vi "Tx Packet Page.vi"(8 "error in (no error)":errorcluster, 11 "Node Ptr":T3 format="%.0x") -> (0 "error out":errorcluster)   [LabVIEW 2019, in "UDP-Custom-Device System Explorer.lvlib"]
uses:
  UDP-Custom-Device System Explorer.lvlib
  Shared/Types/Shared - Transmit Flag Options.ctl
  Shared/Types/Shared - Transmit Echo Options.ctl
  <vilib>/NI VeriStand/Custom Device API/Custom Device Item Ref.ctl
  Types/Page References/Refs - Tx Packets Page.ctl
  Shared/Types/Shared - Channel Data Type.ctl
  <vilib>/NI VeriStand/Custom Device API/Custom Device API.lvlib
  Property Accessors/Tx Packet Accessors.lvlib
  Shared/UDP-Custom-Device Shared.lvlib
  <vilib>/NI VeriStand/Custom Device Tools/Custom Device Utility Library/Custom Device Utility Library.lvlib
  Property Accessors/Shared Packet Accessors.lvlib
  Property Accessors/Tx Channel Accessors.lvlib
  Property Accessors/Tx Channel Section Accessors.lvlib
panel:
  in  "Config Threading":bool
  in  "Debug Mode":bool caption="Auto-Assign Local NIC"
  in  "Transmit Echo Options":T1
  in  "Transmit Options":T2=enum."One-Shot"
  in  "Port as Channel?":bool caption="Auto-Assign Local NIC"
  in  "TTL":u16=1
  in  "Multicast?":bool caption="Auto-Assign Local NIC"
  in  "Channel Config Export":bool
  in  "Configure Header":bool
  in  "Endianness":u16(ring) items=["big-endian"=0, "little-endian"=2]
  in  "Auto-Assign Local NIC":bool
  in  "Port":u16
  in  "IP Address of Local NIC":string
  in  "General Header 3":cluster{"Section Name":string}={"Section Name"="Network Settings"}
  out "Packet ID":i32
  in  "Destination Port":u16
  in  "IP Address of Destination":string
  in  "Description":string
  in  "Name":string
  in  "General Header 2":cluster{"Section Name":string}={"Section Name"="Configured Channels"}
  in  "Tx Channels":i32[](listbox)
  in  "SHDocVw.IWebBrowser":refnum<k7>(container)
  in  "General Header":cluster{"Section Name":string}={"Section Name"="Packet Configuration"}
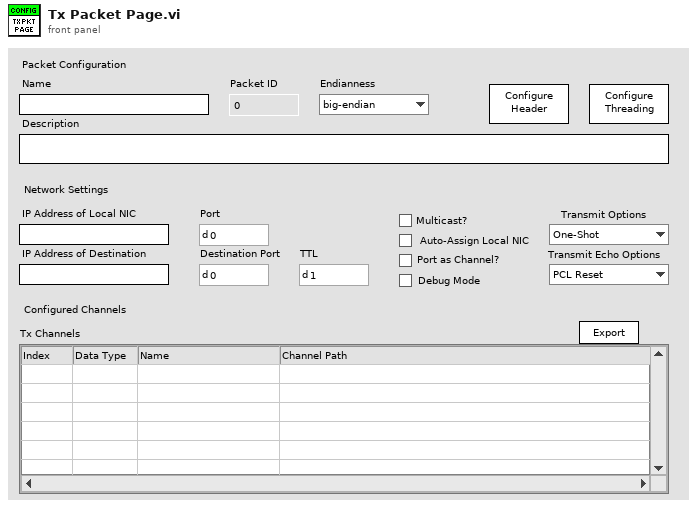
[diagram p1: front panel]
types:
  T1 = typedef "UDP-Custom-Device Shared.lvlib/Shared - Transmit Echo Options.ctl" = enum16{"PCL Reset", "Counter", "Mirror"}
  T2 = typedef "UDP-Custom-Device Shared.lvlib/Shared - Transmit Flag Options.ctl" = enum16{"Always", "One-Shot", "Toggle"}
  T3 = typedef "Custom Device API.lvlib/Custom Device Item Ref.ctl" = u64
  T4 = typedef "UDP-Custom-Device System Explorer.lvlib/Refs - Tx Packets Page.ctl" = cluster{"Tx Channels":refnum<vi>, "Name":refnum<vi>, "Description":refnum<vi>, "Packet ID":refnum<vi>, "Dest IP Address":refnum<vi>, "Dest Port":refnum<vi>, "Source IP Address":refnum<vi>, "Source Port":refnum<vi>, "Auto Assign Local NIC":refnum<vi>, "Endianness":refnum<vi>, "Channel Config Export":refnum<vi>, "TTL":refnum<vi>, "Multicast?":refnum<vi>, "Port as Channel?":refnum<vi>, "Transmit Options":refnum<vi>, "Transmit Echo Options":refnum<vi>, "Debug Mode":refnum<vi>}
  T5 = enum8{"Enabled", "Disabled", "Disabled and Grayed Out"}
  T6 = typedef "UDP-Custom-Device Shared.lvlib/Shared - Channel Data Type.ctl" = enum16{"Boolean", "Single", "Double", "I8", "I16", "I32", "I64", "U8", "U16", "U32", "U64"}
  T7 = typedef "Custom Device API.lvlib/Custom Device Commands.ctl" = enum16{"Default", "Item renamed", "Shutdown", "Dynamic button pressed"}
  T8 = typedef "UDP-Custom-Device System Explorer.lvlib/Thread Configuration.ctl" = cluster{"targetProcessor":i8, "targetPriority":i16, "Synchronization":T9, "loopPeriod":u32, "pclDecimation":u16, "threadManagement":T10}
  T9 = typedef "UDP-Custom-Device System Explorer.lvlib/Thread Sync Reference.ctl" = enum16{"PCL", "Async"}
  T10 = typedef "UDP-Custom-Device Shared.lvlib/Shared - Thread Management.ctl" = enum16{"Untimed (Default)", "Timed (High Priority)"}
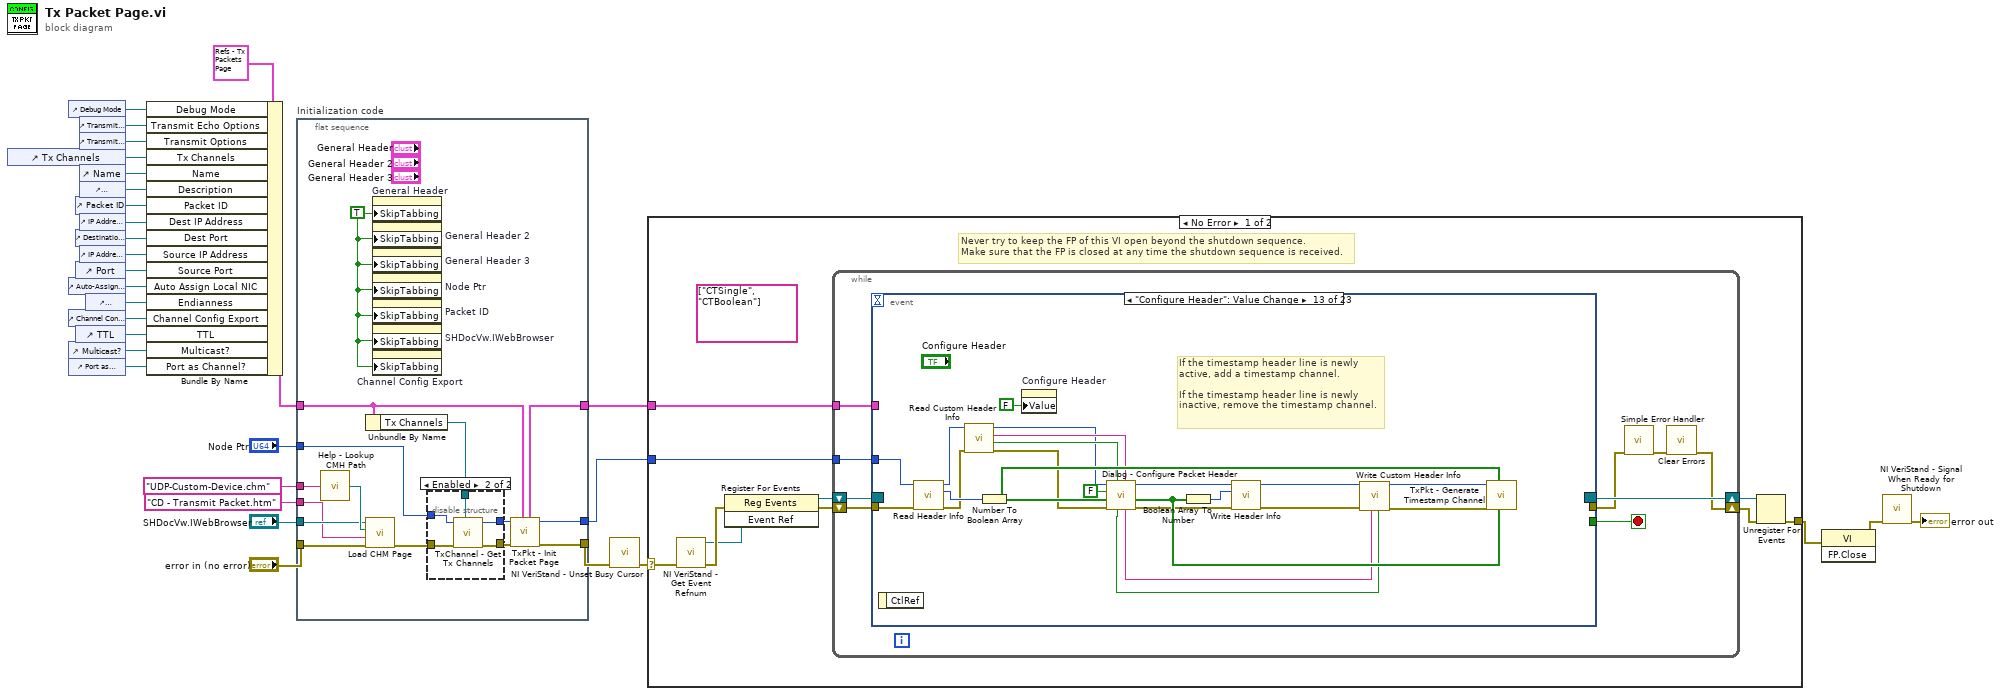
[diagram p0: block diagram]
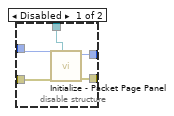
[diagram p2: hidden frame]
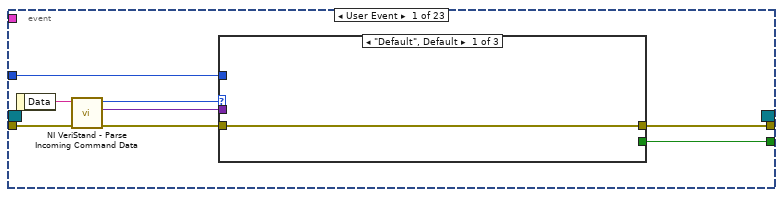
[diagram p3: hidden frame]
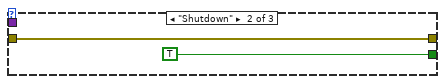
[diagram p4: hidden frame]
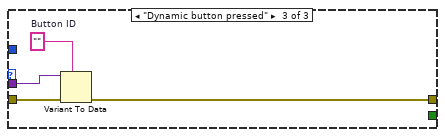
[diagram p5: hidden frame]
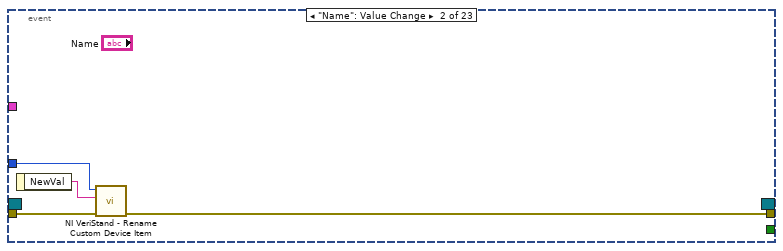
[diagram p6: hidden frame]
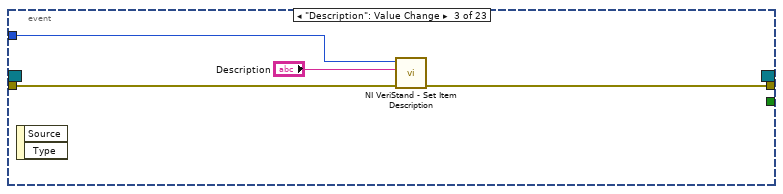
[diagram p7: hidden frame]
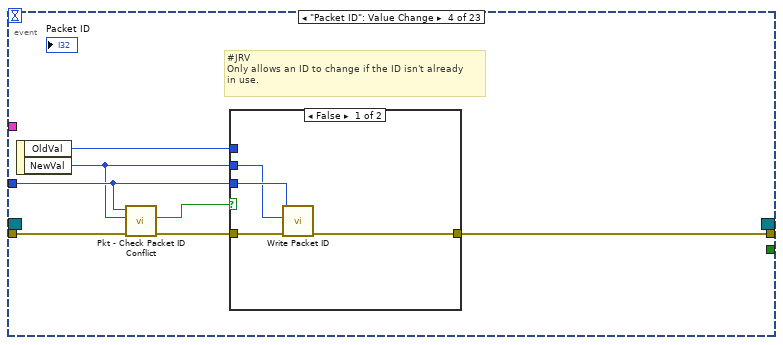
[diagram p8: hidden frame]
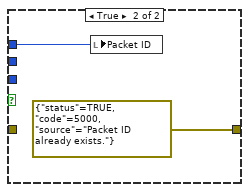
[diagram p9: hidden frame]
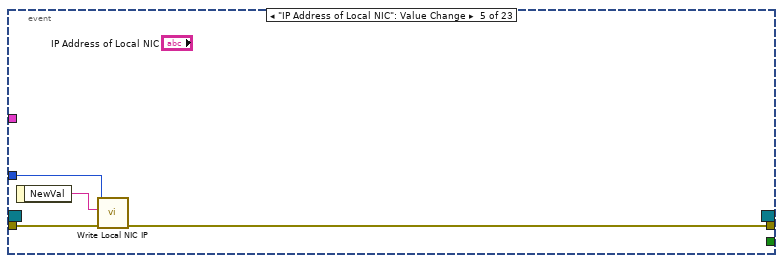
[diagram p10: hidden frame]
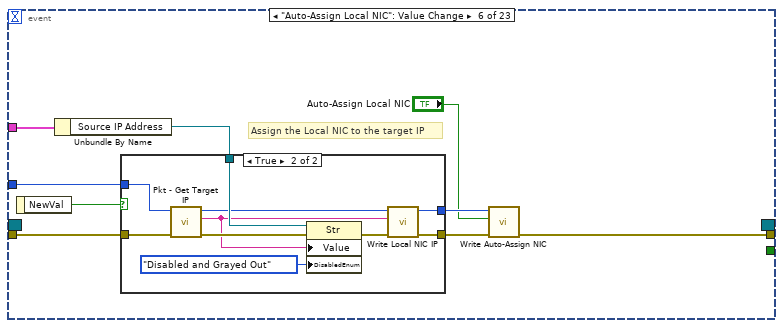
[diagram p11: hidden frame]
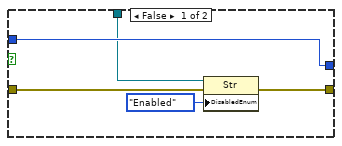
[diagram p12: hidden frame]
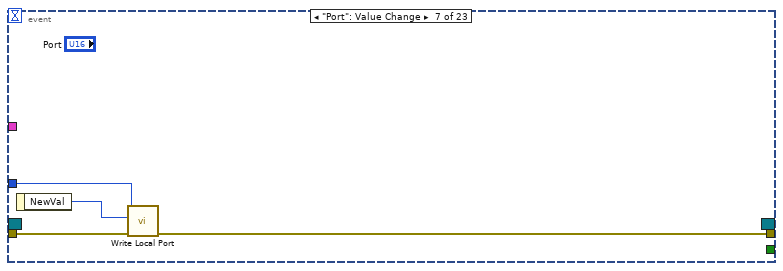
[diagram p13: hidden frame]
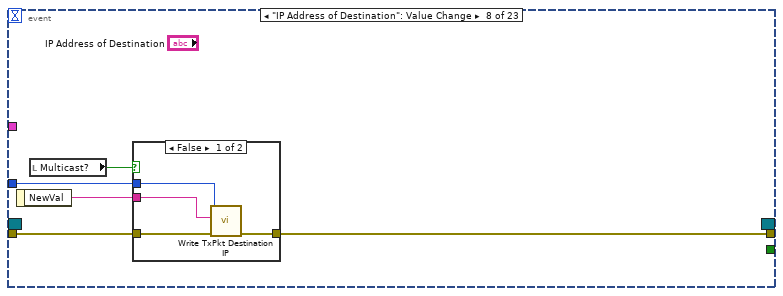
[diagram p14: hidden frame]
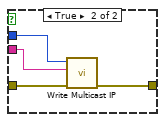
[diagram p15: hidden frame]
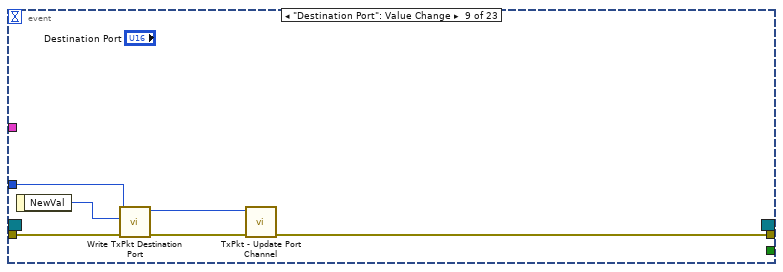
[diagram p16: hidden frame]
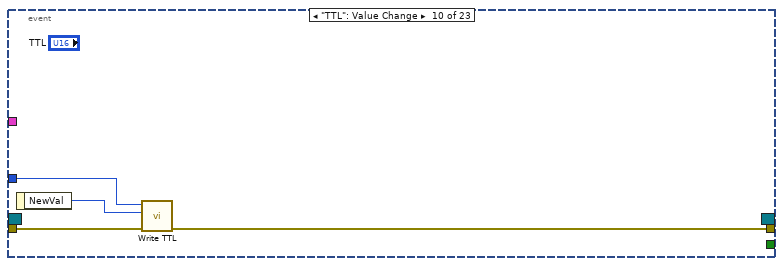
[diagram p17: hidden frame]
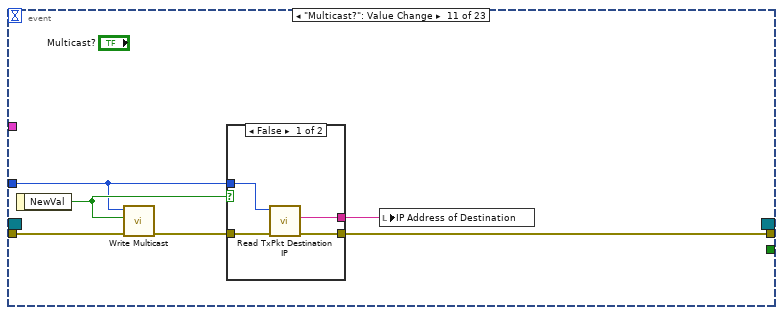
[diagram p18: hidden frame]
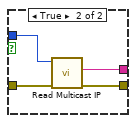
[diagram p19: hidden frame]
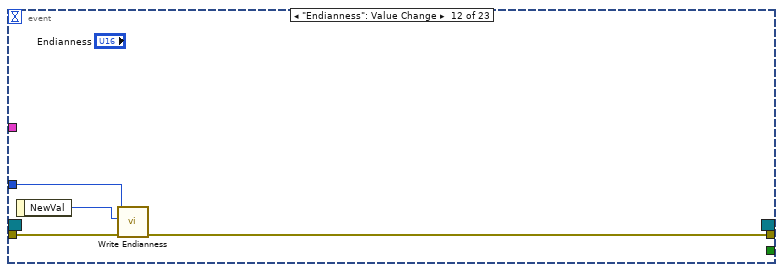
[diagram p20: hidden frame]
diagram:
  n1 = control-ref of="Tx Channels"() -> (w17:refnum<vi>)
  n2 = control-ref of="Debug Mode"() -> (w1:refnum<vi>)
  n3 = control-ref of="Auto-Assign Local NIC"() -> (w10:refnum<vi>)
  n4 = control-ref of="Channel Config Export"() -> (w7:refnum<vi>)
  n5 = control-ref of="Multicast?"() -> (w5:refnum<vi>)
  n6 = control-ref of="Port as Channel?"() -> (w4:refnum<vi>)
  n7 = control-ref of="Packet ID"() -> (w13:refnum<vi>)
  n8 = control-ref of="Destination Port"() -> (w14:refnum<vi>)
  n9 = control-ref of="Port"() -> (w11:refnum<vi>)
  n10 = control-ref of="TTL"() -> (w6:refnum<vi>)
  n11 = control-ref of="Transmit Echo Options"() -> (w2:refnum<vi>)
  n12 = control-ref of="Transmit Options"() -> (w3:refnum<vi>)
  n13 = control-ref of="Name"() -> (w9:refnum<vi>)
  n14 = control-ref of="Description"() -> (w16:refnum<vi>)
  n15 = control-ref of="IP Address of Destination"() -> (w15:refnum<vi>)
  n16 = control-ref of="IP Address of Local NIC"() -> (w12:refnum<vi>)
  n17 = control-ref of="Endianness"() -> (w8:refnum<vi>)
  n18 = Bundle By Name(cluster=T4 {"Tx Channels"=refnum, "Name"=refnum, "Description"=refnum, "Packet ID"=refnum, "Dest IP Address"=refnum, "Dest Port"=refnum, "Source IP Address"=refnum, "Source Port"=refnum, "Auto Assign Local NIC"=refnum, "Endianness"=refnum, "Channel Config Export"=refnum, "TTL"=refnum, "Multicast?"=refnum, "Port as Channel?"=refnum, "Transmit Options"=refnum, "Transmit Echo Options"=refnum, "Debug Mode"=refnum} ("Tx Channels Section Cluster"), "Debug Mode"=w1, "Transmit Echo Options"=w2, "Transmit Options"=w3, "Tx Channels"=w17, "Name"=w9, "Description"=w16, "Packet ID"=w13, "Dest IP Address"=w15, "Dest Port"=w14, "Source IP Address"=w12, "Source Port"=w11, "Auto Assign Local NIC"=w10, "Endianness"=w8, "Channel Config Export"=w7, "TTL"=w6, "Multicast?"=w5, "Port as Channel?"=w4) -> (w20:T4)
  n19 = flat-sequence "Initialization code" {
    tunnel: "error in (no error)" -> [w37]
    tunnel: "Node Ptr" -> [w46]
    tunnel: [w41] -> w27
    tunnel: [w42] -> w24
    tunnel: "SHDocVw.IWebBrowser" -> [w36]
    tunnel: "CD - Transmit Packet.htm" ("CD_CHM_Section") -> [w34]
    tunnel: "UDP-Custom-Device.chm" ("CD_CHM_FileName") -> [w35]
    tunnel: w20 -> [w40]
    tunnel: [w39] -> w19
    frame #0 {
      w32 = TRUE ("Skip When Tabbing")
      n20 = call "Help - Lookup CMH Path.vi"("Main CMH File"=w35) -> ("Compiled CMH Path"=w38:path)
      n21 = Unbundle By Name(w40) -> ("Tx Channels"=w45:refnum<vi>)
      n22 = call <vilib>:"Load CHM Page.vi"("error in (no error)"=w37, "HTML File"=w34, "Compiled CHM Path"=w38, "Web Browser Reference"=w36) -> ("error out"=w33:errorcluster)  [unwired: 7 in]
      n23 = property on="General Header" class="Clust (strict)"("SkipTabbing"=w32) -> ()  [unwired: 2 in, 2 out]
      n24 = property on="General Header 2" class="Clust (strict)"("SkipTabbing"=w32) -> ()  [unwired: 2 in, 2 out]
      n25 = property on="General Header 3" class="Clust (strict)"("SkipTabbing"=w32) -> ()  [unwired: 2 in, 2 out]
      n26 = property on="Node Ptr" class="DigNum (strict)"("SkipTabbing"=w32) -> ()  [unwired: 2 in, 2 out]
      n27 = property on="Packet ID" class="DigNum (strict)"("SkipTabbing"=w32) -> ()  [unwired: 2 in, 2 out]
      n28 = property on="SHDocVw.IWebBrowser" class="AXCont"("SkipTabbing"=w32) -> ()  [unwired: 2 in, 2 out]
      n29 = property on="Channel Config Export" class="Bool"("SkipTabbing"=w32) -> ()  [unwired: 2 in, 2 out]
      n30 = disable-structure shown="Enabled" {
        disable-tunnel: w46 -> [w51 w55]
        disable-tunnel: w45 -> [w50 w54]
        disable-tunnel: [w49 w52] -> w44
        disable-tunnel: [w48 w53] -> w43
        disable-tunnel: w33 -> [w47 w56]
        frame Disabled {
          n31 = call "Initialize - Packet Page Panel.vi"("Channels Listbox"=w50, "error in (no error)"=w47, "Item Ref in"=w51) -> ("error out"=w49:errorcluster, "Item Ref out"=w48:T3)  [unwired: 7 in]
        }
        frame Enabled {
          n32 = call "TxChannel - Get Tx Channels.vi"("MCLB"=w54, "error in (no error)"=w56, "Node Ptr"=w55) -> ("error out"=w52:errorcluster, "Node Ptr out"=w53:T3)  [unwired: 6 in, 1 out]
        }
      }
      n33 = call "TxPkt - Init Packet Page.vi"("Tx Packets Cluster In"=w40, "error in (no error)"=w44, "Node Ptr In"=w43) -> ("error out"=w41:errorcluster, "Node Ptr Out"=w42:T3, "Tx Packets Cluster Out"=w39:T4)  [unwired: 6 in]
    }
  }
  n34 = call <vilib>:"NI VeriStand - Unset Busy Cursor.vi"("error in (no error)"=w27) -> ("error out"=w26:errorcluster)  [unwired: 10 out]
  n35 = case shown="No Error" w26 {
    selector: w26 -> [w58 w343]
    tunnel: [w63 w341] -> w31
    tunnel: w24 -> [w59 _]
    tunnel: w19 -> [w57 _]
    frame No Error {
      (unwired) string[] ["CTSingle", "CTBoolean"] ("item names")
      # "Never try to keep the FP of this VI open beyond the shutdown sequence.\nMake sure that the FP is closed at any time the shutdown sequence is received."
      n36 = call <vilib>:"NI VeriStand - Get Event Refnum.vi"("error in (no error)"=w58) -> ("error out"=w66:errorcluster, "Event Ref"=w62:refnum<user-event>)  [unwired: 9 out]
      n37 = register-events(error in=w66, w62) -> (reference out=w60:refnum<event-registration>, error out=w61:errorcluster)  [unwired: 1 in]
      n38 = while {
        tunnel: w59 -> [w71]
        shift-right: [w68] -> w64
        shift-left: w61 -> [w74]
        shift-right: [w75] -> w65
        shift-left: w60 -> [w73]
        tunnel: w57 -> [w67]
        stop <- w72 stop-if-true
        n39 = event shown="[12] \"Configure Header\": Value Change" {
          selector: w73 -> [_ _ _ _ _ _ _ _ _ _ _ _ _ _ _ _ _ _ _ _ _ _ _]
          dyn-events: [_ _ _ _ _ _ _ _ _ _ _ _ _ _ _ _ _ _ _ _ _ _ _] -> w75
          timeout: _ -> [_ _ _ _ _ _ _ _ _ _ _ _ _ _ _ _ _ _ _ _ _ _ _]
          tunnel: w74 -> [w83 w94 w98 w100 w114 w124 w142 w148 w160 w164 w172 w184 w200 w213 w223 w226 w230 w233 w241 w245 w275 _ w287]
          tunnel: [w79 _ _ _ _ _ _ _ _ _ _ _ _ _ _ _ _ _ _ _ _ _ _] -> w72
          tunnel: [w78 w91 w95 w105 w113 w117 w141 w145 w157 w163 w170 w183 _ w209 w219 w224 w229 w232 w236 w244 w253 _ w286] -> w70
          tunnel: w71 -> [w77 w92 w97 w103 w115 w123 w143 w147 w162 w166 w167 w182 w201 w217 w222 w227 w231 w235 w242 w246 w273 _ w288]
          tunnel: w67 -> [_ _ _ _ _ w122 _ _ _ _ _ _ _ _ _ _ _ _ _ _ w271 _ _]
          event User Event {
            n40 = event-data() -> ("Data"=w82:string)  [unwired: 1 out]
            n41 = call <vilib>:"NI VeriStand - Parse Incoming Command Data.vi"("error in (no error)"=w83, "Incoming data"=w82) -> ("error out"=w81:errorcluster, "Outgoing data"=w76:variant, "Action"=w80:T7)  [unwired: 7 out]
            n42 = case shown="\"Default\", Default" w80 {
              tunnel: w81 -> [w84 w85 w90]
              tunnel: [_ TRUE _] -> w79
              tunnel: [w84 w85 w87] -> w78
              tunnel: w77 -> [_ _ _]
              tunnel: w76 -> [_ _ w89]
              frame "Default", Default {
              }
              frame "Shutdown" {
              }
              frame "Dynamic button pressed" {
                w88 = ""  # Button ID
                n43 = Variant To Data(error in=w90, type=w88, Variant=w89) -> (error out=w87:errorcluster)  [unwired: 1 out]
              }
            }
          }
          event "Name": Value Change {
            n44 = event-data() -> ("NewVal"=w93:string)  [unwired: 1 out]
            n45 = call <vilib>:"NI VeriStand - Rename Custom Device Item.vi"("error in (no error)"=w94, "New Name"=w93, "Item Ref in"=w92) -> ("error out"=w91:errorcluster)  [unwired: 6 in, 2 out]
          }
          event "Description": Value Change {
            n46 = event-data() -> ()  [unwired: 3 out]
            n47 = call <vilib>:"NI VeriStand - Set Item Description.vi"("error in (no error)"=w98, "Description"="Description", "Item Ref in"=w97) -> ("error out"=w95:errorcluster)  [unwired: 6 in, 2 out]
          }
          event "Packet ID": Value Change {
            # "#JRV\nOnly allows an ID to change if the ID isn't already\nin use."
            n48 = event-data() -> ("OldVal"=w104:i32, "NewVal"=w102:i32)  [unwired: 1 out]
            n49 = call "Pkt - Check Packet ID Conflict.vi"("error in (no error)"=w100, "New ID"=w102, "Packet Ref In"=w103) -> ("error out"=w99:errorcluster, "Conflicting ID?"=w101:bool)  [unwired: 7 in]
            n50 = case shown="False" w101 {
              tunnel: w99 -> [w107 _]
              tunnel: w103 -> [w109 _]
              tunnel: [w106 errorcluster {"status"=TRUE, "code"=5000, "source"="Packet ID already exists."} ("error out")] -> w105
              tunnel: w104 -> [_ w111]
              tunnel: w102 -> [w108 _]
              frame False {
                n51 = call "Write Packet ID.vi"("error in (no error)"=w107, "Packet ID"=w108, "Node Ptr"=w109) -> ("error out"=w106:errorcluster)  [unwired: 7 in, 1 out]
              }
              frame True {
                n52 = local write "Packet ID"(w111) -> ()
              }
            }
          }
          event "IP Address of Local NIC": Value Change {
            n53 = event-data() -> ("NewVal"=w112:string)  [unwired: 1 out]
            n54 = call "Write Local NIC IP.vi"("error in (no error)"=w114, "IP Address of Local NIC"=w112, "Node Ptr"=w115) -> ("error out"=w113:errorcluster)  [unwired: 7 in, 1 out]
          }
          event "Auto-Assign Local NIC": Value Change {
            # "Assign the Local NIC to the target IP"
            n55 = event-data() -> ("NewVal"=w121:bool)  [unwired: 1 out]
            n56 = Unbundle By Name(w122) -> ("Source IP Address"=w120:refnum<vi>)
            n57 = case shown="True" w121 {
              tunnel: w124 -> [w129 w137]
              tunnel: [w127 w131] -> w118
              tunnel: [w126 w130] -> w119
              tunnel: w123 -> [w126 w136]
              tunnel: w120 -> [w125 w135]
              frame False {
                n58 = property class="Str"(reference=w125, error in=w129, "DisabledEnum"=T5."Enabled" ("Disabled")) -> (error out=w127:errorcluster)  [unwired: 1 out]
              }
              frame True {
                n59 = call "Pkt - Get Target IP.vi"("error in"=w137, "Item Ref in"=w136) -> ("error out"=w139:errorcluster, "IPAddress"=w133:string, "Item Ref out"=w134:T3)  [unwired: 7 in]
                n60 = property class="Str"(reference=w135, error in=w139, "Value"=w133, "DisabledEnum"=T5."Disabled and Grayed Out" ("Disabled")) -> (error out=w132:errorcluster)  [unwired: 1 out]
                n61 = call "Write Local NIC IP.vi"("error in (no error)"=w132, "IP Address of Local NIC"=w133, "Node Ptr"=w134) -> ("error out"=w131:errorcluster, "Node Ptr out"=w130:T3)  [unwired: 7 in]
              }
            }
            n62 = call "Write Auto-Assign NIC.vi"("error in (no error)"=w118, "Auto-Assign NIC"="Auto-Assign Local NIC", "Node Ptr"=w119) -> ("error out"=w117:errorcluster)  [unwired: 7 in, 1 out]
          }
          event "Port": Value Change {
            n63 = event-data() -> ("NewVal"=w140:u16)  [unwired: 1 out]
            n64 = call "Write Local Port.vi"("error in (no error)"=w142, "Port"=w140, "Node Ptr"=w143) -> ("error out"=w141:errorcluster)  [unwired: 7 in, 1 out]
          }
          event "IP Address of Destination": Value Change {
            n65 = event-data() -> ("NewVal"=w146:string)  [unwired: 1 out]
            n66 = local read "Multicast?"() -> (w144:bool)
            n67 = case shown="False" w144 {
              tunnel: w148 -> [w152 w154]
              tunnel: w147 -> [w151 w156]
              tunnel: w146 -> [w150 w155]
              tunnel: [w149 w153] -> w145
              frame False {
                n68 = call "Write TxPkt Destination IP.vi"("error in (no error)"=w152, "Destination IP"=w150, "Node Ptr"=w151) -> ("error out"=w149:errorcluster)  [unwired: 7 in, 1 out]
              }
              frame True {
                n69 = call "Write Multicast IP.vi"("error in (no error)"=w154, "Multicast IP Address"=w155, "Node Ptr"=w156) -> ("error out"=w153:errorcluster)  [unwired: 7 in, 1 out]
              }
            }
          }
          event "Destination Port": Value Change {
            n70 = event-data() -> ("NewVal"=w161:u16)  [unwired: 1 out]
            n71 = call "Write TxPkt Destination Port.vi"("error in (no error)"=w160, "Destination Port"=w161, "Node Ptr"=w162) -> ("error out"=w158:errorcluster, "Node Ptr out"=w159:T3)  [unwired: 7 in]
            n72 = call "TxPkt - Update Port Channel.vi"("error in (no error)"=w158, "Packet Ref in"=w159) -> ("error out"=w157:errorcluster)  [unwired: 8 in, 1 out]
          }
          event "TTL": Value Change {
            n73 = event-data() -> ("NewVal"=w165:u16)  [unwired: 1 out]
            n74 = call "Write TTL.vi"("error in (no error)"=w164, "TTL"=w165, "Node Ptr"=w166) -> ("error out"=w163:errorcluster)  [unwired: 7 in, 1 out]
          }
          event "Multicast?": Value Change {
            n75 = event-data() -> ("NewVal"=w169:bool)  [unwired: 1 out]
            n76 = call "Write Multicast.vi"("error in (no error)"=w172, "Multicast"=w169, "Node Ptr"=w167) -> ("error out"=w171:errorcluster)  [unwired: 7 in, 1 out]
            n77 = case shown="False" w169 {
              tunnel: w171 -> [w175 w180]
              tunnel: [w173 w179] -> w170
              tunnel: [w174 w178] -> w168
              tunnel: w167 -> [w176 w177]
              frame False {
                n78 = call "Read TxPkt Destination IP.vi"("error in (no error)"=w175, "Node Ptr"=w176) -> ("error out"=w173:errorcluster, "Destination IP"=w174:string)  [unwired: 7 in, 1 out]
              }
              frame True {
                n79 = call "Read Multicast IP.vi"("error in (no error)"=w180, "Node Ptr"=w177) -> ("error out"=w179:errorcluster, "Multicast IP Address"=w178:string)  [unwired: 7 in, 1 out]
              }
            }
            n80 = local write "IP Address of Destination"(w168) -> ()
          }
          event "Endianness": Value Change {
            n81 = event-data() -> ("NewVal"=w181:u16)  [unwired: 1 out]
            n82 = call "Write Endianness.vi"("error in (no error)"=w184, "Endianness"=w181, "Node Ptr"=w182) -> ("error out"=w183:errorcluster)  [unwired: 7 in, 1 out]
          }
          event "Configure Header": Value Change {
            # "If the timestamp header line is newly\nactive, add a timestamp channel.\n\nIf the timestamp header line is newly\ninactive, remove the timestamp channel."
            n83 = event-data() -> ()  [unwired: 2 out]
            n84 = call "Read Header Info.vi"("error in (no error)"=w200, "Node Ptr"=w201) -> ("error out"=w197:errorcluster, "Header Info"=w199:u32, "Node Ptr out"=w196:T3)  [unwired: 7 in]
            n85 = call "Read Custom Header Info.vi"("error in (no error)"=w197, "Node Ptr"=w196) -> ("error out"=w195:errorcluster, "CustomHeaderEnabled"=w194:bool, "CustomHeaderLogicProfile"=w193:string, "Node Ptr out"=w192:T3)  [unwired: 6 in]
            n86 = Number To Boolean Array(number=w199) -> (Boolean array=w206:bool[])
            n87 = property on="Configure Header" class="Bool (strict)"("Value"=FALSE ("Configure Header")) -> ()  [unwired: 2 in, 2 out]
            n88 = call "Dialog - Configure Packet Header.vi"("CustomHeaderLogicProfile"=w193, "CustomHeaderEnabled 2"=w194, "error in (no error)"=w195, "Header Elements In"=w206, "HideCustomHeder"=FALSE, "Packet Ref in"=w192) -> ("error out"=w203:errorcluster, "Header Elements Out"=w205:bool[], "Packet Ref out"=w204:T3, "Custom Heather Logic"=w191:string, "CustomHeaderEnabled"=w190:bool)  [unwired: 1 in]
            n89 = Boolean Array To Number(Boolean array=w205) -> (number=w202:u32)
            n90 = call "Write Header Info.vi"("error in (no error)"=w203, "Header Info"=w202, "Node Ptr"=w204) -> ("error out"=w189:errorcluster, "Node Ptr out"=w188:T3)  [unwired: 7 in]
            n91 = call "Write Custom Header Info.vi"("CustomHeatherEnabled"=w190, "HeatherCustomLogic"=w191, "error in (no error)"=w189, "Node Ptr"=w188) -> ("error out"=w187:errorcluster, "Node Ptr out"=w186:T3)  [unwired: 6 in]
            n92 = call "TxPkt - Generate Timestamp Channel.vi"("New Header Config"=w205, "Previous Header Config"=w206, "error in (no error)"=w187, "Packet Ref in"=w186) -> ()  [unwired: 6 in, 2 out]
          }
          event "Config Threading": Value Change {
            # "Dialog for managing the threading\noptions for the timed structures"
            n93 = event-data() -> ()  [unwired: 5 out]
            n94 = call "ThreadCfg - Read TxPkt Config.vi"("error in (no error)"=w213, "Node Ptr In"=w217) -> ("error out"=w214:errorcluster, "threadOptions"=w215:T8, "Node Ptr Out"=w216:T3)  [unwired: 7 in]
            n95 = call "Dialog - Configure Threading.vi"("rxPacket?"=FALSE, "error in (no error)"=w214, "threadOptions in"=w215, "Packet Ref in"=w216) -> ("error out"=w210:errorcluster, "threadOptions out"=w211:T8, "Packet Ref out"=w212:T3)  [unwired: 4 in]
            n96 = call "ThreadCfg - Write TxPkt Config.vi"("error in (no error)"=w210, "threadOptions"=w211, "Node Ptr In"=w212) -> ("error out"=w209:errorcluster)  [unwired: 7 in, 1 out]
            n97 = property on="Config Threading" class="Bool (strict)"("Value"=FALSE ("Config Threading")) -> ()  [unwired: 2 in, 2 out]
          }
          event "Port as Channel?": Value Change {
            n98 = event-data() -> ("NewVal"=w221:bool)  [unwired: 1 out]
            n99 = call "Write TxPkt Port as Channel.vi"("error in (no error)"=w223, "Port as Channel"=w221, "Node Ptr"=w222) -> ("error out"=w220:errorcluster, "Node Ptr out"=w218:T3)  [unwired: 7 in]
            n100 = call "TxPkt - Handle Port Channel.vi"("error in (no error)"=w220, "Packet Ref in"=w218) -> ("error out"=w219:errorcluster)  [unwired: 8 in, 1 out]
          }
          event Value Change {
            n101 = event-data() -> ("NewVal"=w225:T2)  [unwired: 1 out]
            n102 = call "Write TxPkt Transmit Option.vi"("error in (no error)"=w226, "Transmit Options"=w225, "Node Ptr"=w227) -> ("error out"=w224:errorcluster)  [unwired: 7 in, 1 out]
          }
          event Value Change {
            n103 = event-data() -> ("NewVal"=w228:T1)  [unwired: 1 out]
            n104 = call "Write TxPkt Transmit Echo Option.vi"("error in (no error)"=w230, "Transmit Echo Options"=w228, "Node Ptr"=w231) -> ("error out"=w229:errorcluster)  [unwired: 7 in, 1 out]
          }
          event "Debug Mode": Value Change {
            n105 = event-data() -> ("NewVal"=w234:bool)  [unwired: 1 out]
            n106 = call "Write Debug Mode.vi"("error in (no error)"=w233, "Debug Mode"=w234, "Node Ptr"=w235) -> ("error out"=w232:errorcluster)  [unwired: 7 in, 1 out]
          }
          event "Channel Config Export": Value Change {
            n107 = event-data() -> ()  [unwired: 2 out]
            n108 = property on="Channel Config Export" class="Bool"(error in=w241, "DisabledEnum"=T5."Disabled and Grayed Out" ("Disabled")) -> (error out=w240:errorcluster)  [unwired: 1 in, 1 out]
            n109 = call "TxPkt - Export Channel Configuration.vi"("error in (no error)"=w240, "Packet Ref in"=w242) -> ("error out"=w237:errorcluster)  [unwired: 8 in, 1 out]
            n110 = property on="Channel Config Export" class="Bool"(error in=w237, "DisabledEnum"=T5."Enabled" ("Disabled")) -> (error out=w236:errorcluster)  [unwired: 1 in, 1 out]
          }
          event "Tx Channels": Value Change {
            n111 = event-data() -> ()  [unwired: 2 out]
            n112 = property on="Tx Channels" class="MCListbox (strict)"() -> ("ItemNames"=w247:string[][], "Value"=w248:i32[])  [unwired: 2 in, 2 out]
            n113 = for {
              tunnel: w247 -> [w252]
              tunnel: [w251] -> w243 mode=indexing
              tunnel: w248 -> [w250] mode=indexing
              n114 = Index Array(array=w252, index (row)=w250, index (col)=2 ("disabled index (row)")) -> (element=w251:string)
            }
            n115 = call "Write Selected Channels.vi"("error in (no error)"=w245, "Selected Channel Names"=w243, "Node Ptr"=w246) -> ("error out"=w244:errorcluster)  [unwired: 7 in, 1 out]
          }
          event "Tx Channels": Drag Ended {
            n116 = event-data() -> ()  [unwired: 2 out]
            n117 = Unbundle By Name(w271) -> ("Tx Channels"=w267:refnum<vi>)
            n118 = property class="MCListbox (strict)"(reference=w267, error in=w275) -> (error out=w274:errorcluster, "ItemNames"=w264:string[][])  [unwired: 1 out]
            n119 = Index Array(array=w264, index (col)=0 ("disabled index (col)")) -> (element=w266:string[])  [unwired: 1 in]
            n120 = Array Size(array=w266) -> (size(s)=w265:i32)
            n121 = for {
              N: w265 -> [_]
              tunnel: [w276] -> w262 mode=indexing
              i -> [w278]
              n122 = Number To Decimal String(number=w278, width (-)=i16 3) -> (decimal integer string=w276:string)
            }
            n123 = Index Array(array=w264, index (col) #1=2 ("index (row)"), index (col) #2=3 ("index (col)"), index (col) #3=1 ("index (col)")) -> (element #1=w257:string[], element #2=w272:string[], element #3=w259:string[])  [unwired: 3 in]
            n124 = Replace Array Subset(array=w264, new element=w262, index (col)=0 ("disabled index (col)")) -> (w261:string[][])  [unwired: 1 in]
            n125 = call "TxPkt - Update Properties.vi"("Channel Data Types"=w259, "error in (no error)"=w274, "Channel Paths"=w272, "Channel Names"=w257, "Item Ref in"=w273) -> ("error out"=w256:errorcluster, "Item Ref out"=w258:T3)  [unwired: 5 in]
            n126 = property class="MCListbox (strict)"(reference=w267, "ItemNames"=w261) -> ()  [unwired: 1 in, 2 out]
            n127 = call "Write Selected Channels.vi"("error in (no error)"=w256, "Selected Channel Names"=w257, "Node Ptr"=w258) -> ("error out"=w255:errorcluster, "Node Ptr out"=w254:T3)  [unwired: 7 in]
            n128 = call "TxChannel - Update Tx Channel Order.vi"("error in (no error)"=w255, "Node Ptr"=w254) -> ("error out"=w253:errorcluster)  [unwired: 8 in, 1 out]
          }
          event "Tx Channels": Shortcut Menu Activation? {
            n129 = event-data() -> ("MenuRef"=w283:refnum<k9>)  [unwired: 1 out]
            n130 = Insert Menu Items(7:string[] ["RemoveChannels", "ChangeType"] ("item names"), 8:string[] ["Remove Channels", "Change Type"] ("item names"), 9:w283) -> (3:w281:refnum<k9>)  [unwired: 3 in, 2 out]
            n131 = call "Pkt - Menu Data Types.vi"() -> ("Menu Tags"=w279:string[], "Menu Names"=w280:string[])  [unwired: 10 in]
            n132 = Insert Menu Items(5:"ChangeType", 7:w279, 8:w280, 9:w281) -> ()  [unwired: 2 in, 3 out]
            n133 = event-data() -> ()  [unwired: 2 in, 1 out]
          }
          event "Tx Channels": Shortcut Menu Selection (User) {
            n134 = event-data() -> ("ItemTag"=w289:string)  [unwired: 1 out]
            n135 = case shown="Default" w289 {
              selector: w289 -> [_ w320]
              tunnel: w288 -> [w296 w306]
              tunnel: w287 -> [w295 w307]
              tunnel: [w290 w309] -> w286
              frame "RemoveChannels" {
                n136 = property on="Tx Channels" class="MCListbox (strict)"() -> ("ItemNames"=w294:string[][], "Value"=w293:i32[])  [unwired: 2 in, 2 out]
                n137 = call "RTM - Remove Channels.vi"("error in (no error)"=w295, "Node Ptr In"=w296) -> ("error out"=w290:errorcluster)  [unwired: 9 in]
                n138 = for {
                  tunnel: w293 -> [w300]
                  tunnel: [w301] -> w292 mode=indexing if=w297
                  tunnel: w294 -> [w301] mode=indexing
                  i -> [w299]
                  n139 = Search 1D Array(1D array=w300, element=w299) -> (index of element=w298:i32)  [unwired: 1 in]
                  n140 = Less Than 0?(x=w298) -> (x < 0?=w297:bool)
                }
                n141 = property on="Tx Channels" class="MCListbox (strict)"("ItemNames"=w292, "Value"=i32[] [] ("Tx Channels")) -> ()  [unwired: 2 in, 2 out]
              }
              frame Default {
                n142 = case shown="\"CTBoolean\"" w320 {
                  tunnel: [Shared_-_Channel_Data_Type."Single" ("Data Type") Shared_-_Channel_Data_Type."Double" ("Data Type") Shared_-_Channel_Data_Type."Boolean" ("Data Type") Shared_-_Channel_Data_Type."I8" ("Data Type") Shared_-_Channel_Data_Type."I16" ("Data Type") Shared_-_Channel_Data_Type."I32" ("Data Type") Shared_-_Channel_Data_Type."I64" ("Data Type") Shared_-_Channel_Data_Type."U8" ("Data Type") Shared_-_Channel_Data_Type."U16" ("Data Type") Shared_-_Channel_Data_Type."U32" ("Data Type") Shared_-_Channel_Data_Type."U64" ("Data Type")] -> w318
                  frame "CTSingle", Default {
                  }
                  frame "CTDouble" {
                  }
                  frame "CTBoolean" {
                  }
                  frame "CTI8" {
                  }
                  frame "CTI16" {
                  }
                  frame "CTI32" {
                  }
                  frame "CTI64" {
                  }
                  frame "CTU8" {
                  }
                  frame "CTU16" {
                  }
                  frame "CTU32" {
                  }
                  frame "CTU64" {
                  }
                }
                n143 = local read "Tx Channels"() -> (w317:i32[])
                n144 = call <vilib>:"NI VeriStand - Get Item Reference by Name.vi"("error in (no error)"=w307, "Item Name"="Channels" ("Section Name"), "Parent Ref in"=w306) -> ("error out"=w304:errorcluster, "Item Ref"=w305:T3)  [unwired: 5 in, 2 out]
                n145 = call "Read Tx Channel Dependent Nodes.vi"("error in (no error)"=w304, "Node Ptr"=w305) -> ("error out"=w303:errorcluster, "Dependent Node Refs"=w302:T3[])  [unwired: 7 in, 1 out]
                n146 = call "Read TxPkt Data Types.vi"("error in (no error)"=w303, "Node Ptr"=w306) -> ("error out"=w316:errorcluster, "Data types"=w319:T6[], "Node Ptr out"=w315:T3)  [unwired: 7 in]
                n147 = for {
                  tunnel: w318 -> [w322]
                  tunnel: w317 -> [w326] mode=indexing
                  tunnel: [w324] -> w312
                  tunnel: w316 -> [w325]
                  shift-right: [w329] -> w314
                  shift-left: w319 -> [w327]
                  shift-right: [w328] -> w313
                  shift-left: w315 -> [w328]
                  tunnel: w302 -> [w321]
                  n148 = Index Array(array=w321, index=w326) -> (element=w323:T3)
                  n149 = Replace Array Subset(array=w327, new element=w322, index=w326) -> (w329:T6[])
                  n150 = call "Write Tx Data Type.vi"("error in (no error)"=w325, "Data Type"=w322, "Node Ptr"=w323) -> ("error out"=w324:errorcluster)  [unwired: 6 in, 2 out]
                }
                n151 = call "Write TxPkt Data Types.vi"("error in (no error)"=w312, "Data Types"=w314, "Node Ptr"=w313) -> ("error out"=w310:errorcluster, "Node Ptr out"=w311:T3)  [unwired: 7 in]
                n152 = call <vilib>:"NI VeriStand - Highlight Node in System Explorer.vi"("error in (no error)"=w310, "Item Ref in"=w311) -> ("error out"=w309:errorcluster)  [unwired: 8 in, 1 out]
              }
            }
          }
        }
        n153 = call <vilib>:"Simple Error Handler.vi"("error in (no error)"=w70) -> ("error out"=w69:errorcluster)  [unwired: 1 in, 7 out]
        n154 = call <vilib>:"Clear Errors.vi"("error in (no error)"=w69) -> ("error out"=w68:errorcluster)  [unwired: 1 in, 5 out]
      }
      n155 = Unregister For Events(event registration refnum=w65, error in=w64) -> (error out=w63:errorcluster)
    }
    frame Error {
      n156 = call <vilib>:"Simple Error Handler.vi"("error in (no error)"=w343) -> ("error out"=w342:errorcluster)  [unwired: 1 in, 7 out]
      n157 = call <vilib>:"Clear Errors.vi"("error in (no error)"=w342) -> ("error out"=w341:errorcluster)  [unwired: 1 in, 5 out]
    }
  }
  n158 = invoke class="VI" method="FP.Close"(error in=w31) -> (error out=w30:errorcluster)  [unwired: 2 in, 2 out]
  n159 = call <vilib>:"NI VeriStand - Signal When Ready for Shutdown.vi"("error in (no error)"=w30) -> ("error out"=→"error out":errorcluster)  [unwired: 10 out]
